vi "FPGA_lock-in_generat-light.vi"() -> ()   [LabVIEW 2013]
uses:
  fast cycles/FPGA_run-states.ctl
  <vilib>/rvi/Emulation/niFpgaSctlEmulationGetInTimedLoop.vi
  <vilib>/rvi/Emulation/niFpgaEmulationReportErrorSimple.vi
  <vilib>/rvi/Emulation/niFpgaGetClockAttributes.vi
  <vilib>/rvi/FIFO/Fifo_Resource/nirvififoEmulationReadFpgaImpl.vi
  <vilib>/rvi/DataTransferAndStorage/Container/Common/niFpgaContainerGetUniqueNameForEmu.vi
  <vilib>/rvi/Emulation/niFpgaProcessEmulError.vi
  <vilib>/rvi/Emulation/niFpgaCriticalErrorInLSC.vi
  <vilib>/rvi/FIFO/Fifo_Resource/nirvififoEmulationWriteFpgaImpl.vi
  <vilib>/rvi/Memory/Memory_Emulation/nirvimemoryEmulation.vi
  <vilib>/rvi/Memory/Memory_Emulation/nirvimemoryFastEmulation.vi
  <vilib>/rvi/Memory/Memory_Emulation/niFpgaMemoryEmulationCacheClearOnFirstRun.vi
  <vilib>/rvi/Memory/Memory_Emulation/nirvimemoryEmulationManagerCache_MakeExclusive.vi
  <vilib>/rvi/Memory/Memory_Emulation/niFpgaMemoryEmulationValidateCache.vi
  <vilib>/rvi/Memory/Memory_Emulation/nirvimemoryEmulationManagerCache_ReleaseExclusive.vi
  <vilib>/rvi/Memory/Memory_Emulation/nirvimemoryEmulationManagerCache_InsertValue.vi
  <vilib>/Utility/error.llb/Clear Errors.vi
  <vilib>/rvi/Memory/Memory_Emulation/nirvimemoryEmulationManagerCache_GetValue.vi
  <vilib>/rvi/Memory/Memory_Emulation/nirvimemoryEmulationManagerCache_SetValue.vi
  <vilib>/rvi/Emulation/niFpgaSctlEmulationResourceMgr.vi
  <vilib>/rvi/eio/common/nirviEmuTemplateMethod_errors.vi
  <vilib>/rvi/DataTransferAndStorage/Container/XNode/niFpgaContainer.xnode
  <vilib>/rvi/FIFO/Fifo_Resource/nirvififoEmulationRead.vi
  <vilib>/rvi/FIFO/Fifo_Resource/nirvififoEmulationWrite.vi
  <vilib>/eio/EIONode/EIONode.xnode
panel:
  in  "DAC mem adr":u8
  out "LI channel":u16
  in  "inhibate lock-in":bool=TRUE
  in  "clock reset":bool
  in  "clock divider":u32=20
  in  "Amplitude":fxp<+/-,16,16>
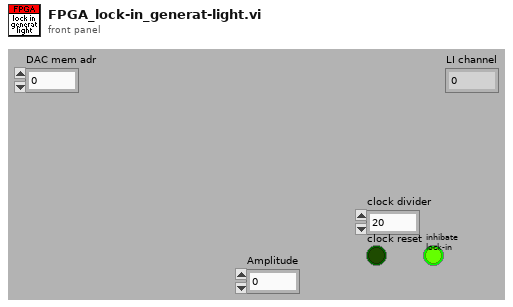
[diagram p1: front panel]
types:
  T1 = typedef "FPGA_run-states.ctl" = enum16{"stopped", "check", "reserve", "run", "release"}
  T2 = cluster{"Boolean array[0]":bool, "Boolean array[1]":bool}
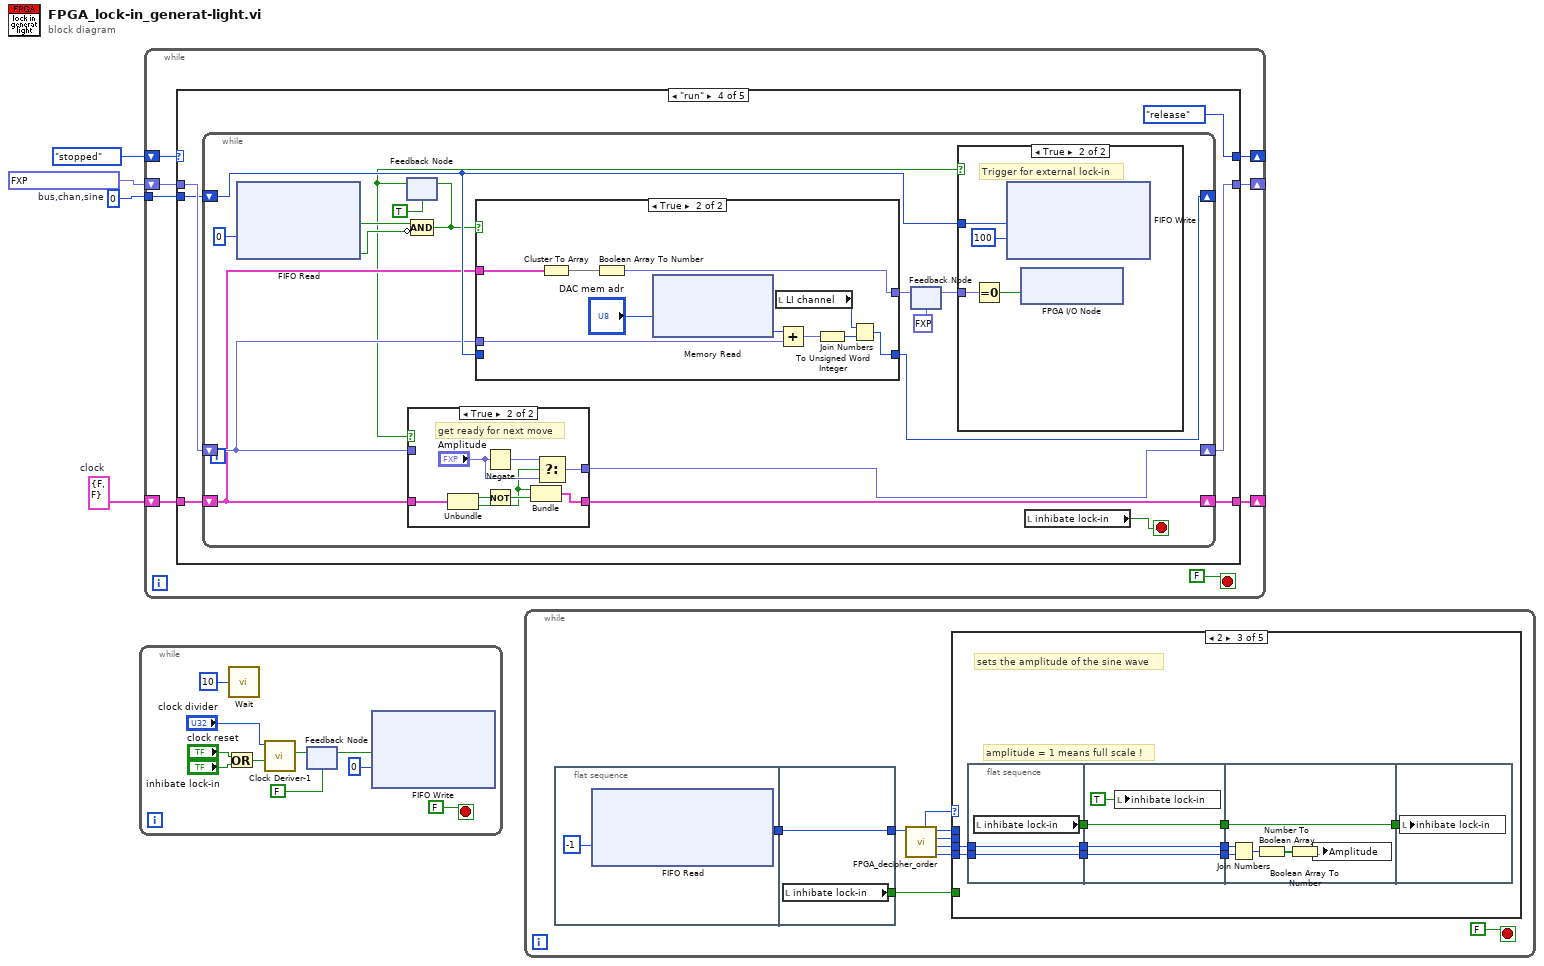
[diagram p0: block diagram]
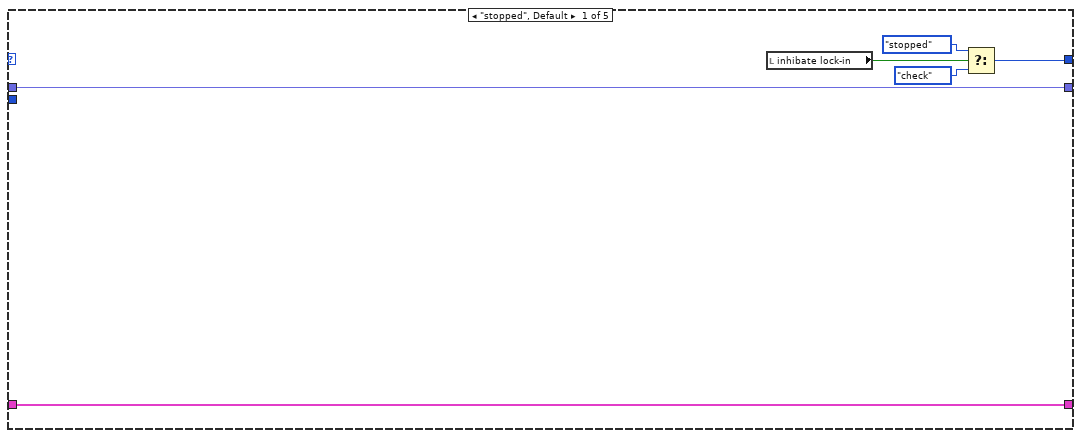
[diagram p2: hidden frame]
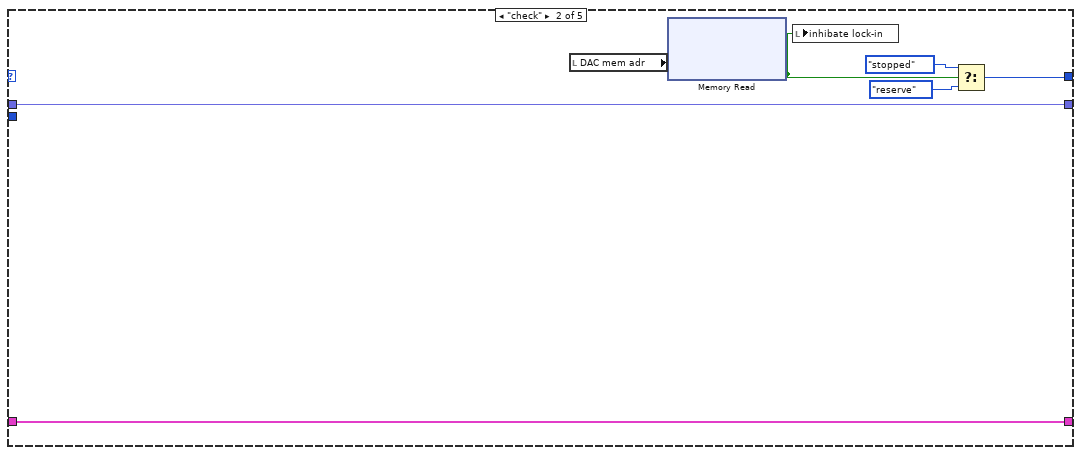
[diagram p3: hidden frame]
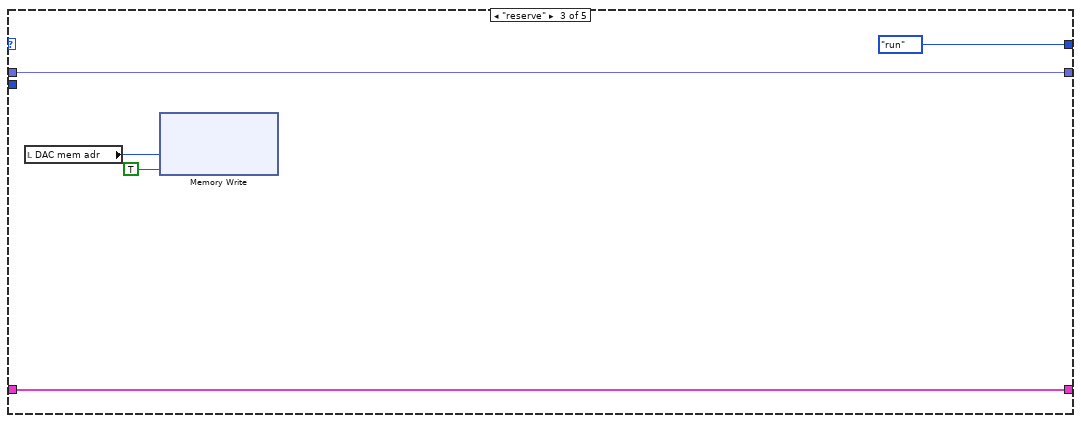
[diagram p4: hidden frame]
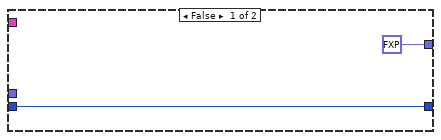
[diagram p7: hidden frame]
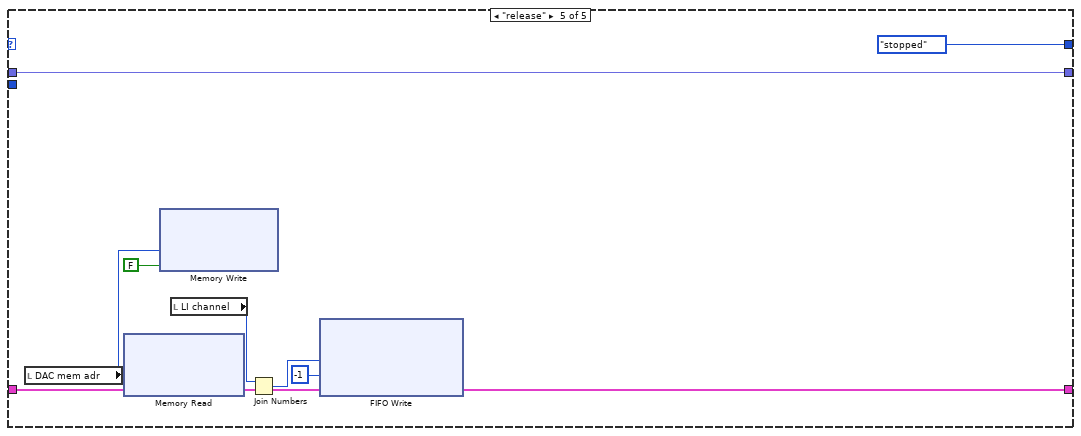
[diagram p8: hidden frame]
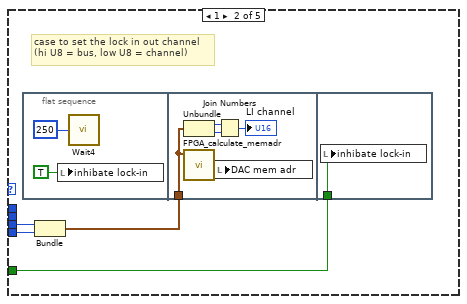
[diagram p10: hidden frame]
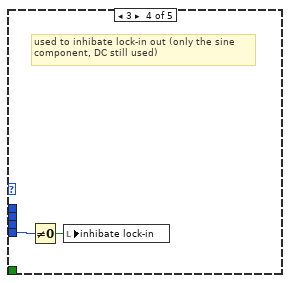
[diagram p11: hidden frame]
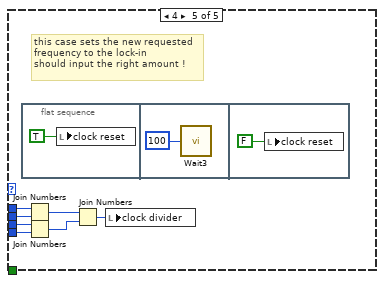
[diagram p12: hidden frame]
diagram:
  w2 = u32 0  # bus,chan,sine
  w3 = T2 {"Boolean array[0]"=FALSE, "Boolean array[1]"=FALSE}  # clock
  n1 = while {
    stop <- FALSE stop-if-true
    n2 = Or(x="clock reset", y="inhibate lock-in") -> (x .or. y?=w11:bool)
    n3 = call "Wait"("Count(uSec)"=u8 10 ("Count(Ticks)")) -> ()  [unwired: 1 out]
    n4 = call "Clock Deriver-1.vi"("Reset"=w11, "Divisor"="clock divider") -> ("Clock Out"=w9:bool)  [unwired: 9 out]
    n5 = feedback-in #1(w9) -> ()
    n6 = feedback #1(FALSE ("Clock Out")) -> (w6:bool)
    n7 = xnode ("FIFO Write")("Element"=w6, "Timeout"=0) -> ()  [unwired: 1 in, 2 out]
  }
  n8 = while {
    shift-right: [w19] -> _
    shift-left: w3 -> [w21]
    shift-right: [w18] -> _
    shift-left: fxp<+/-,16,16> 0.0 ("Amplitude") -> [w22]
    tunnel: w2 -> [w20]
    shift-right: [w16] -> _
    shift-left: FPGA_run-states."stopped" ("run states") -> [w17]
    stop <- FALSE stop-if-true
    n9 = case shown="\"run\"" w17 {
      tunnel: w22 -> [w24 w30 w37 w46 w96]
      tunnel: w21 -> [w23 w31 w36 w45 w95]
      tunnel: w20 -> [_ _ _ w44 _]
      tunnel: [w23 w31 w36 w43 w95] -> w19
      tunnel: [w24 w30 w37 w42 w96] -> w18
      tunnel: [w25 w32 FPGA_run-states."run" ("run states") FPGA_run-states."release" ("run states") FPGA_run-states."stopped" ("run states")] -> w16
      frame "stopped", Default {
        n10 = local read "inhibate lock-in"() -> (w28:bool)
        n11 = Select(t=FPGA_run-states."stopped" ("run states"), s=w28, f=FPGA_run-states."check" ("run states")) -> (s? t:f=w25:T1)
      }
      frame "check" {
        n12 = local read "DAC mem adr"() -> (w35:u8)
        n13 = xnode ("Memory Read")("Address"=w35) -> ("Data"=w29:bool)  [unwired: 1 in, 1 out]
        n14 = local write "inhibate lock-in"(w29) -> ()
        n15 = Select(t=FPGA_run-states."stopped" ("run states"), s=w29, f=FPGA_run-states."reserve" ("run states")) -> (s? t:f=w32:T1)
      }
      frame "reserve" {
        n16 = local read "DAC mem adr"() -> (w40:u8)
        n17 = xnode ("Memory Write")("Address"=w40, "Data"=TRUE) -> ()  [unwired: 1 in, 1 out]
      }
      frame "run" {
        n18 = while {
          shift-right: [w62] -> _
          shift-left: w44 -> [w60]
          shift-right: [w51] -> w43
          shift-left: w45 -> [w50]
          shift-right: [w55] -> w42
          shift-left: w46 -> [w54]
          stop <- w49 stop-if-true
          n19 = xnode ("FIFO Read")("Timeout"=0) -> ("Element"=w59:bool, "Timed Out?"=w57:bool)  [unwired: 1 in, 1 out]
          n20 = feedback #2(TRUE) -> (w47:bool)
          n21 = case shown="True" w47 {
            tunnel: [w64 w72] -> w55
            tunnel: w54 -> [w64 _]
            tunnel: w50 -> [w63 w70]
            tunnel: [w63 w65] -> w51
            frame False {
            }
            frame True {
              # "get ready for next move"
              n22 = Unbundle(w70) -> ("Boolean array[0]"=w68:bool, "Boolean array[1]"=w66:bool)
              n23 = Negate ("Opposé")(x="Amplitude") -> (-x=w71:fxp<+/-,16,16>)
              n24 = Not(x=w68) -> (.not. x?=w67:bool)
              n25 = Bundle("Boolean array[1]"=w66, w67) -> (w65:cluster{"Boolean array[1]":bool, bool})  [unwired: 1 out]
              n26 = Select(t=w71, s=w66, f="Amplitude") -> (s? t:f=w72:fxp<+/-,16,16>)
            }
          }
          n27 = Compound Arithmetic op=AND(w59, invert w57) -> (w48:bool)
          n28 = feedback-in #2(w48) -> ()
          n29 = case shown="True" w48 {
            tunnel: [w78 w85] -> w62
            tunnel: [fxp<+,2,2> 0.0 ("mem adr") w81] -> w61
            tunnel: w60 -> [w78 _]
            tunnel: w54 -> [_ w80]
            tunnel: w50 -> [_ w83]
            frame False {
            }
            frame True {
              n30 = Cluster To Array(cluster=w83) -> (array=w82:bool[])
              n31 = Boolean Array To Number(Boolean array=w82) -> (number=w81:fxp<+,2,2>)
              n32 = xnode ("Memory Read")("Address"="DAC mem adr") -> ("Data"=w79:u16)  [unwired: 1 in, 1 out]
              n33 = local read "LI channel"() -> (w87:u16)
              n34 = Add(x=w79, y=w80) -> (x+y=w88:fxp<+,16,16>)
              n35 = To Unsigned Word Integer(number=w88) -> (unsigned 16bit integer=w86:u16)
              n36 = Join Numbers(hi=w87, lo=w86) -> ((hi.lo)=w85:u32)
            }
          }
          n37 = feedback-in #3(w61) -> ()
          n38 = feedback #3(fxp<+,2,2> 0.0 ("mem adr")) -> (w53:fxp<+,2,2>)
          n39 = case shown="True" w47 {
            tunnel: w60 -> [_ w75]
            tunnel: w53 -> [_ w73]
            frame False {
            }
            frame True {
              # "Trigger for external lock-in"
              n40 = Equal To 0?(x=w73) -> (x = 0?=w74:bool)
              n41 = xnode ("FIFO Write")("Element"=w75, "Timeout"=100) -> ()  [unwired: 1 in, 2 out]
              n42 = xnode "FPGA I/O Node"("Port0/DIO0"=w74) -> ()  [unwired: 1 in, 1 out]
            }
          }
          n43 = local read "inhibate lock-in"() -> (w49:bool)
        }
      }
      frame "release" {
        n44 = local read "DAC mem adr"() -> (w93:u8)
        n45 = xnode ("Memory Read")("Address"=w93) -> ("Data"=w91:u16)  [unwired: 1 in, 1 out]
        n46 = xnode ("Memory Write")("Address"=w93, "Data"=FALSE) -> ()  [unwired: 1 in, 1 out]
        n47 = local read "LI channel"() -> (w94:u16)
        n48 = Join Numbers(hi=w94, lo=w91) -> ((hi.lo)=w90:u32)
        n49 = xnode ("FIFO Write")("Element"=w90, "Timeout"=-1) -> ()  [unwired: 1 in, 2 out]
      }
    }
  }
  n50 = while {
    stop <- FALSE stop-if-true
    n51 = flat-sequence {
      tunnel: [w107] -> w99
      tunnel: [w110] -> w105
      tunnel: w99 -> [w110]
      tunnel: [w109] -> w98
      frame #0 {
        n52 = xnode ("FIFO Read")("Timeout"=-1) -> ("Element"=w107:u64)  [unwired: 1 in, 2 out]
      }
      frame #1 {
        n53 = local read "inhibate lock-in"() -> (w109:bool)
      }
    }
    n54 = call "FPGA_decipher_order.vi"("order in"=w105) -> ("data 1"=w103:u8, "data 2"=w102:u8, "data 3"=w101:u8, "data 4"=w100:u8, "order out"=w104:u8)  [unwired: 6 out]
    n55 = case shown="2" w104 {
      tunnel: w103 -> [_ w113 w130 w147 w151]
      tunnel: w102 -> [_ w114 w131 _ w152]
      tunnel: w101 -> [_ _ _ _ w153]
      tunnel: w100 -> [_ _ _ _ w154]
      tunnel: w98 -> [_ w111 _ _ _]
      frame 0, Default {
      }
      frame 1 {
        # "case to set the lock in out channel\n(hi U8 = bus, low U8 = channel)"
        n56 = flat-sequence {
          tunnel: w112 -> [w120]
          tunnel: w111 -> [w122]
          frame #0 {
            n57 = local write "inhibate lock-in"(TRUE ("inhibate lock-in")) -> ()
            n58 = call "Wait4"("Count(uSec)"=u8 250) -> ()  [unwired: 1 out]
          }
          frame #1 {
            n59 = Unbundle(w120) -> ("data 2"=w118:u8, "data 1"=w119:u8)
            n60 = call "FPGA_calculate_memadr.vi"("Cluster"=w120) -> ("mem adr"=w121:u8)  [unwired: 10 out]
            n61 = Join Numbers(hi=w118, lo=w119) -> ((hi.lo)=→"LI channel":u16)
            n62 = local write "DAC mem adr"(w121) -> ()
          }
          frame #2 {
            n63 = local write "inhibate lock-in"(w122) -> ()
          }
        }
        n64 = Bundle("data 2"=w114, "data 1"=w113) -> (w112:cluster{"data 2":u8, "data 1":u8})  [unwired: 1 out]
      }
      frame 2 {
        # "amplitude = 1 means full scale !"
        # "sets the amplitude of the sine wave"
        n65 = flat-sequence {
          tunnel: w131 -> [w132]
          tunnel: w130 -> [w133]
          tunnel: [w134] -> w127
          tunnel: [w133] -> w126
          tunnel: [w132] -> w123
          tunnel: [w137] -> w128
          tunnel: w127 -> [w137]
          tunnel: w126 -> [w136]
          tunnel: [w136] -> w125
          tunnel: [w135] -> w124
          tunnel: w123 -> [w135]
          tunnel: [w144] -> w129
          tunnel: w128 -> [w144]
          tunnel: w125 -> [w140]
          tunnel: w124 -> [w139]
          tunnel: w129 -> [w145]
          frame #0 {
            n66 = local read "inhibate lock-in"() -> (w134:bool)
          }
          frame #1 {
            n67 = local write "inhibate lock-in"(TRUE ("inhibate lock-in")) -> ()
          }
          frame #2 {
            n68 = Join Numbers(hi=w139, lo=w140) -> ((hi.lo)=w143:u16)
            n69 = Number To Boolean Array(number=w143) -> (Boolean array=w141:bool[])
            n70 = Boolean Array To Number(Boolean array=w141) -> (number=w142:fxp<+/-,16,16>)
            n71 = local write "Amplitude"(w142) -> ()
          }
          frame #3 {
            n72 = local write "inhibate lock-in"(w145) -> ()
          }
        }
      }
      frame 3 {
        # "used to inhibate lock-in out (only the sine\ncomponent, DC still used)"
        n73 = Not Equal To 0?(x=w147) -> (x != 0?=w146:bool)
        n74 = local write "inhibate lock-in"(w146) -> ()
      }
      frame 4 {
        # "this case sets the new requested\nfrequency to the lock-in\nshould input the right amount !"
        n75 = flat-sequence {
          frame #0 {
            n76 = local write "clock reset"(TRUE ("clock reset")) -> ()
          }
          frame #1 {
            n77 = call "Wait3"("Count(uSec)"=u8 100) -> ()  [unwired: 1 out]
          }
          frame #2 {
            n78 = local write "clock reset"(FALSE ("clock reset")) -> ()
          }
        }
        n79 = Join Numbers(hi=w154, lo=w153) -> ((hi.lo)=w150:u16)
        n80 = Join Numbers(hi=w152, lo=w151) -> ((hi.lo)=w149:u16)
        n81 = Join Numbers(hi=w150, lo=w149) -> ((hi.lo)=w148:u32)
        n82 = local write "clock divider"(w148) -> ()
      }
    }
  }
